vi "Instrument Configure Call.vi"(3 "error in":errorcluster, 4 "Instrument Prop In":T1={"Public"={"Column Name"=[], "Trace Color"=[]}, "Private"={"Path"=path "", "VI Refnum"=refnum, "Name"="", "# of Values"=0, "Scale Factors"=[], "Display"=[], "Offset"=[1.0]}} {"Private"."Offset" format="%^_3e"; "Private"."Scale Factors" format="%^_3e"}) -> (0 "error out":errorcluster, 1 "Instrument Prop Out":T1={"Public"={"Column Name"=[], "Trace Color"=[]}, "Private"={"Path"=path "", "VI Refnum"=refnum, "Name"="", "# of Values"=0, "Scale Factors"=[], "Display"=[], "Offset"=[1.0]}} {"Private"."Offset" format="%^_3e"; "Private"."Scale Factors" format="%^_3e"})   [LabVIEW 2024]
uses:
  Sub Controls/Instrument Properties.ctl
  Sub Controls/Public.ctl
  Sub Controls/Private.ctl
  Sub Controls/Instrument Ref.ctl
  Sub Controls/SystemCheckBox-resize.ctl
  Sub Controls/Instrument Actions.ctl
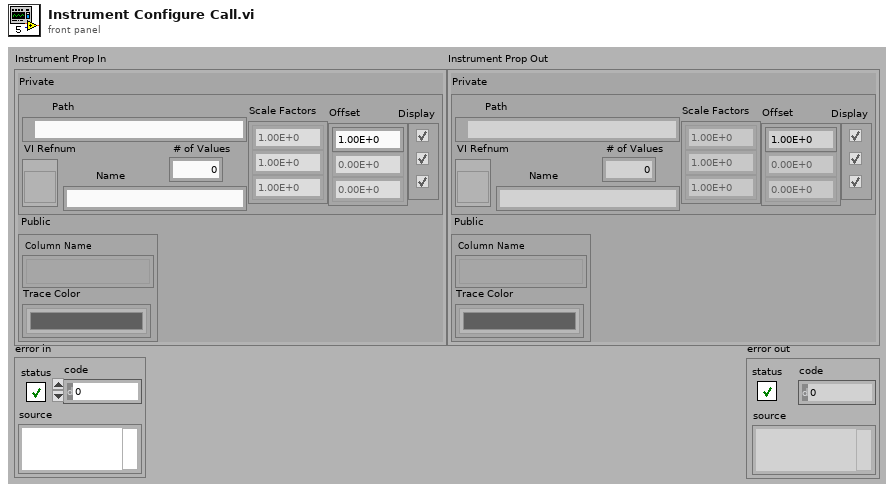
[diagram p1: front panel]
types:
  T1 = typedef "Instrument Properties.ctl" = cluster{"Public":T2, "Private":T3}
  T2 = typedef "Public.ctl" = cluster{"Column Name":string[], "Trace Color":u32[]}
  T3 = typedef "Private.ctl" = cluster{"Path":path, "VI Refnum":T4, "Name":string, "# of Values":i32, "Scale Factors":dbl[], "Display":T5[], "Offset":dbl[]}
  T4 = typedef "Instrument Ref.ctl" = refnum<vi>
  T5 = typedef "SystemCheckBox-resize.ctl" = bool
  T6 = typedef "Instrument Actions.ctl" = enum16{"Scan", "Identify", "New", "Configure", "Initialize", "Test", "Read", "Close"}
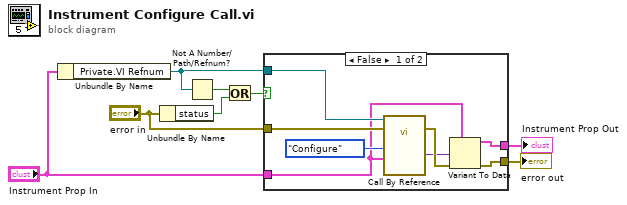
[diagram p0: block diagram]
diagram:
  n1 = Unbundle By Name("Instrument Prop In") -> ("Private.VI Refnum"=w1:T4)
  n2 = Unbundle By Name("error in") -> ("status"=w3:bool)
  n3 = Not A Number/Path/Refnum?(number/path/refnum=w1) -> (NaN/Path/Refnum?=w8:bool)
  n4 = Or(x=w8, y=w3) -> (x .or. y?=w4:bool)
  n5 = case shown="False" w4 {
    tunnel: "error in" -> [w16 w17]
    tunnel: w1 -> [w14 _]
    tunnel: [w11 w18] -> w7
    tunnel: [w10 w17] -> w6
    tunnel: "Instrument Prop In" -> [w9 w18]
    frame False {
      n6 = call-by-ref "?"(reference=w14, error in=w16, "Action"=Instrument_Actions."Configure", "Parameters"=w9) -> (error out=w13:errorcluster, "Output"=w12:variant)  [unwired: 4 in, 2 out]
      n7 = Variant To Data(error in=w13, type=w9, Variant=w12) -> (data=w11:T1, error out=w10:errorcluster)
    }
    frame True {
    }
  }
  "error out" <- w6
  "Instrument Prop Out" <- w7
